vi "detect network devices.vi"(11 "device class":T1={"cDAQ"=TRUE, "cRIO"=TRUE, "Ethernet RIO"=TRUE, "sbRIO"=TRUE, "PXI"=FALSE, "CVS"=FALSE, "Desktop"=FALSE, "FieldPoint"=FALSE, "<No Device Class>"=FALSE}) -> (2 "passed?":bool)   [LabVIEW 2014, in "tests.lvlib"]
uses:
  tests.lvlib
  classes/Device/device class selection.ctl
  classes/Device/FG action.ctl
  classes/Device/Device.lvclass
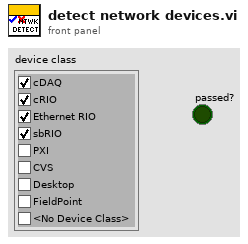
[diagram p1: front panel]
types:
  T1 = typedef "SMI.lvlib/Device.lvclass/device class selection.ctl" = cluster{"cDAQ":bool, "cRIO":bool, "Ethernet RIO":bool, "sbRIO":bool, "PXI":bool, "CVS":bool, "Desktop":bool, "FieldPoint":bool, "<No Device Class>":bool}
  T2 = typedef "SMI.lvlib/Device.lvclass/FG action.ctl" = enum16{"get", "set"}
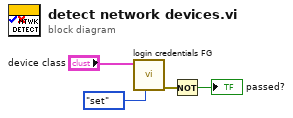
[diagram p0: block diagram]
diagram:
  n1 = call "login credentials FG.vi"("FG action"=FG_action."set", "device class"="device class") -> ("error out"=w3:errorcluster)  [unwired: 8 in, 1 out]
  n2 = Not(x=w3) -> (.not. x?=→"passed?":bool)
